vi "Create AO waveforms.vi"(9 "sampling info":cluster{"Fs":dbl, "#s":dbl}={"Fs"=1000.0, "#s"=1000.0} {"Fs" format="%.2p"}, 10 "reset signal":bool, 11 "Cluster":T1={"amplitude (V)"=[0.001, 2e-08, 0.001, 0.001, 0.001, 2e-08, 0.0, 0.0], "DC (V)"=[0.0, 0.0, 0.0, 0.0, 0.0, 0.0, 0.0, 0.0], "f (Hz)"=[13.0, 13.0, 13.0, 13.0, 13.0, 13.0, 13.0, 13.0], "phase (deg)"=[0.0, 0.0, 0.0, 0.0, 0.0, 0.0, 0.0, 0.0], "demod f (Hz)"=[13.0, 13.0, 13.0, 13.0, 13.0, 13.0, 13.0, 13.0], "function"=[enum."Sine Wave", enum."Sine Wave", enum."Sine Wave", enum."Sine Wave", enum."Sine Wave", enum."Sine Wave", enum."Sine Wave", enum."Sine Wave"]} {"DC (V)" format="%#_6p"; "amplitude (V)" format="%#_6p"}) -> (1 "AO Array":waveform(dbl)[](array[waveform]), 3 "Cluster 2":T1={"amplitude (V)"=[0.001, 2e-08, 0.001, 0.001, 0.001, 2e-08, 0.0, 0.0], "DC (V)"=[0.0, 0.0, 0.0, 0.0, 0.0, 0.0, 0.0, 0.0], "f (Hz)"=[13.0, 13.0, 13.0, 13.0, 13.0, 13.0, 13.0, 13.0], "phase (deg)"=[0.0, 0.0, 0.0, 0.0, 0.0, 0.0, 0.0, 0.0], "demod f (Hz)"=[13.0, 13.0, 13.0, 13.0, 13.0, 13.0, 13.0, 13.0], "function"=[enum."Sine Wave", enum."Sine Wave", enum."Sine Wave", enum."Sine Wave", enum."Sine Wave", enum."Sine Wave", enum."Sine Wave", enum."Sine Wave"]} {"DC (V)" format="%#_6p"; "amplitude (V)" format="%#_6p"})   [LabVIEW 2013]
uses:
  <vilib>/measure/NI_MABase.lvlib
panel:
  out "Waveform Graph":waveform(dbl)[](graph)
  out "Waveform Chart":T2(graph)
  out "phase out":dbl[](array[numeric])
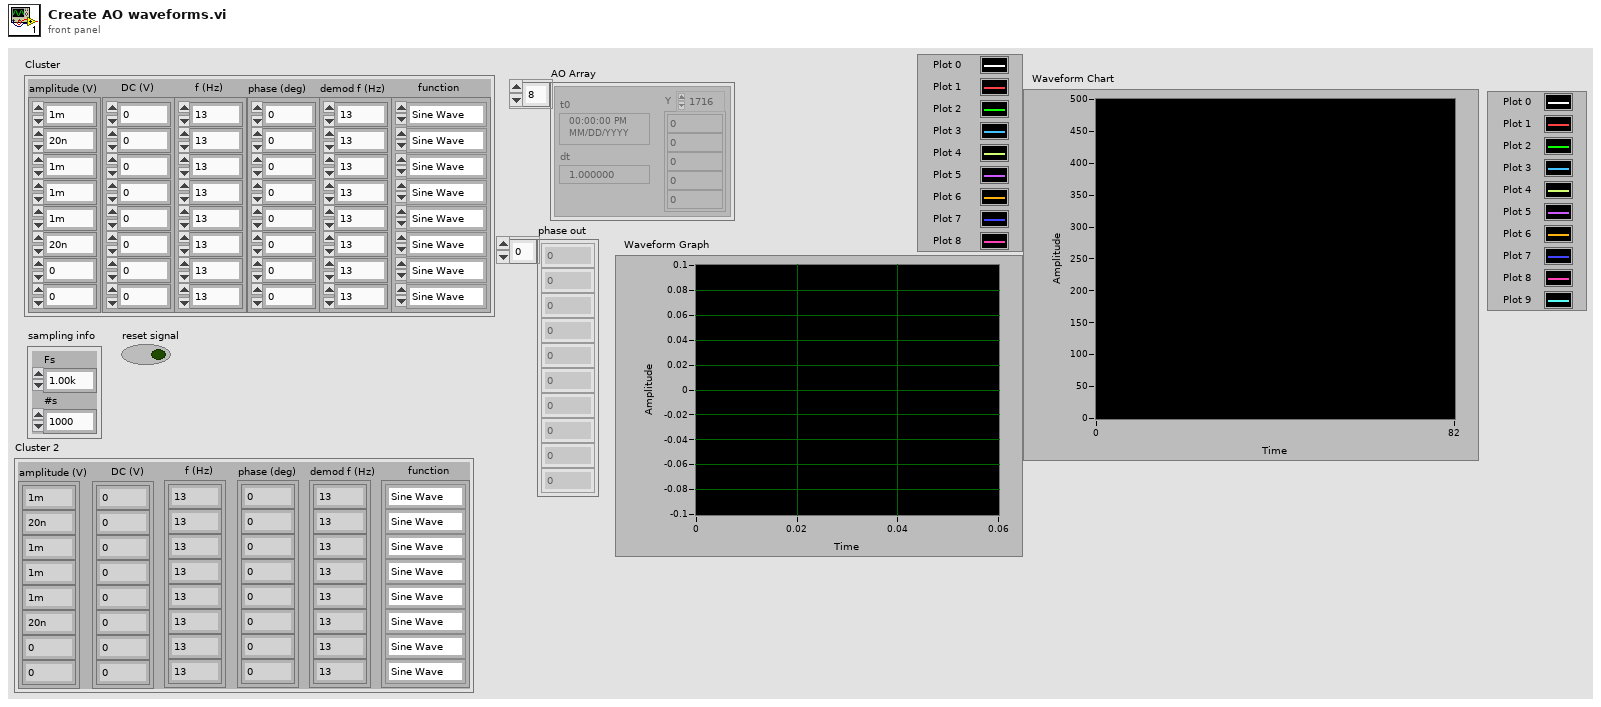
[diagram p1: front panel]
types:
  T1 = cluster{"amplitude (V)":dbl[], "DC (V)":dbl[], "f (Hz)":dbl[], "phase (deg)":dbl[], "demod f (Hz)":dbl[], "function":enum16{"Sine Wave", "Triangle Wave", "Square Wave", "Sawtooth Wave"}[]}
  T2 = cluster{"[0]":dbl, "[1]":dbl, "[2]":dbl, "[3]":dbl, "[4]":dbl, "[5]":dbl, "[6]":dbl, "[7]":dbl, "[8]":dbl}
  T3 = enum16{"Sine Wave", "Triangle Wave", "Square Wave", "Sawtooth Wave"}[]
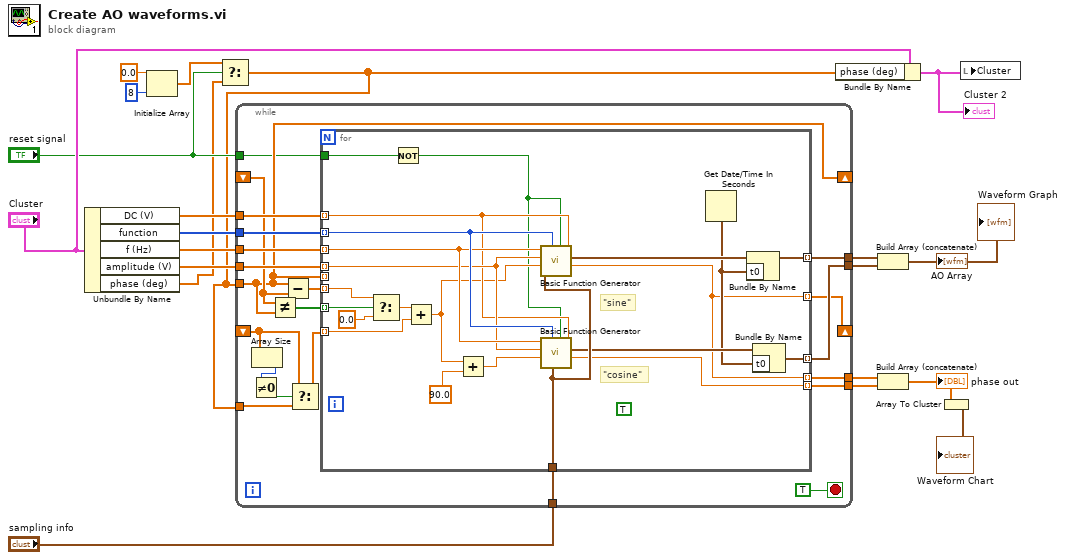
[diagram p0: block diagram]
diagram:
  n1 = Unbundle By Name("Cluster") -> ("DC (V)"=w19:dbl[], "function"=w20:T3, "f (Hz)"=w15:dbl[], "amplitude (V)"=w16:dbl[], "phase (deg)"=w4:dbl[])
  n2 = Initialize Array(0.0 ("element"), 8 ("dimension size")) -> (w6:dbl[])
  n3 = Select(t=w6, s="reset signal", f=w4) -> (s? t:f=w3:dbl[])
  n4 = while {
    tunnel: w20 -> [w41]
    tunnel: w19 -> [w40]
    tunnel: "sampling info" -> [w39]
    tunnel: [w38] -> w1
    tunnel: [w37] -> w17
    tunnel: w16 -> [w36]
    tunnel: w3 -> [w28]
    tunnel: w15 -> [w35]
    tunnel: [w33] -> w13
    tunnel: [w32] -> w14
    shift-right: [w28] -> _
    shift-left: _ -> [w30]
    shift-right: [w27] -> _
    shift-left: _ -> [w22]
    tunnel: w3 -> [w23]
    tunnel: "reset signal" -> [w21]
    stop <- TRUE stop-if-true
    n5 = Array Size(array=w22) -> (size(s)=w25:i32)
    n6 = Not Equal To 0?(x=w25) -> (x != 0?=w24:bool)
    n7 = Not Equal?(x=w30, y=w28) -> (x != y?=w31:bool[])
    n8 = Subtract(x=w28, y=w30) -> (x-y=w29:dbl[])
    n9 = Select(t=w22, s=w24, f=w23) -> (s? t:f=w26:dbl[])
    n10 = for {
      tunnel: w41 -> [w63] mode=indexing
      tunnel: w35 -> [w62] mode=indexing
      tunnel: w36 -> [w61] mode=indexing
      tunnel: w40 -> [w60] mode=indexing
      tunnel: [w57] -> w38 mode=indexing
      tunnel: w39 -> [w59]
      tunnel: [w56] -> w37 mode=indexing
      tunnel: [w51] -> w32 mode=indexing
      tunnel: [w53] -> w33 mode=indexing
      tunnel: w31 -> [w44] mode=indexing
      tunnel: w29 -> [w48] mode=indexing
      tunnel: w28 -> [_] mode=indexing
      tunnel: [w51] -> w27 mode=indexing
      tunnel: w26 -> [w49] mode=indexing
      tunnel: w21 -> [w43]
      (unwired) TRUE
      # "\"cosine\""
      # "\"sine\""
      n11 = Select(t=w48, s=w44, f=0.0) -> (s? t:f=w50:dbl)
      n12 = Not(x=w43) -> (.not. x?=w42:bool)
      n13 = Add(x=w50, y=w49) -> (x+y=w45:dbl)
      n14 = Add(x=w45, y=90.0) -> (x+y=w46:dbl)
      n15 = call <vilib>:"Basic Function Generator.vi"("offset"=w60, "reset signal"=w42, "sampling info"=w59, "signal type"=w63, "phase"=w45, "amplitude"=w61, "frequency"=w62) -> ("phase out"=w51:dbl, "signal out"=w58:waveform(dbl))  [unwired: 2 in, 1 out]
      n16 = call <vilib>:"Basic Function Generator.vi"("offset"=w60, "reset signal"=w42, "sampling info"=w59, "signal type"=w63, "phase"=w46, "amplitude"=w61, "frequency"=w62) -> ("phase out"=w53:dbl, "signal out"=w55:waveform(dbl))  [unwired: 2 in, 1 out]
      n17 = Get Date/Time In Seconds() -> (seconds since 1Jan1904=w54:timestamp)
      n18 = Bundle By Name(cluster=w58, "t0"=w54) -> (w57:waveform(dbl))
      n19 = Bundle By Name(cluster=w55, "t0"=w54) -> (w56:waveform(dbl))
    }
  }
  n20 = Bundle By Name(cluster="Cluster", "phase (deg)"=w3) -> (w9:T1)
  "Cluster 2" <- w9
  n21 = Build Array (concatenate)(w1, w17) -> (→"AO Array" →"Waveform Graph":waveform(dbl)[])
  n22 = Build Array (concatenate)(w14, w13) -> (w12:dbl[])
  "phase out" <- w12
  n23 = Array To Cluster(array=w12) -> (cluster=→"Waveform Chart":T2)
  n24 = local write "Cluster"(w9) -> ()
